vi "End Unpolled Mode.vi"(8 "error in":errorcluster, 11 "Neph in":refnum<class "Nephelometer.lvclass">) -> (0 "error out":errorcluster, 3 "Neph out":refnum<class "Nephelometer.lvclass">)   [LabVIEW 2014, in "Nephelometer.lvclass"]
uses:
  Nephelometer.lvclass
  Reusable/Session APIs/Serial/Serial Session.lvclass
  Nephelometer.lvclass/Nephelometer.ctl
  Accessors/Read Session Handle.vi
  <userlib>/_Session Fwk/Session - Root.lvclass
panel:
  out "Read - Asynchronous":string
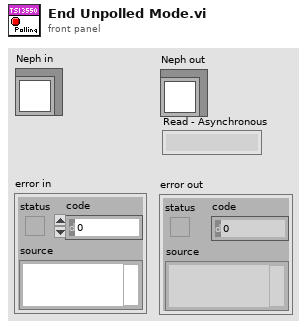
[diagram p1: front panel]
types:
  T1 = typedef "Session - Root.lvclass/Session Handle.ctl" = refnum<data-value>
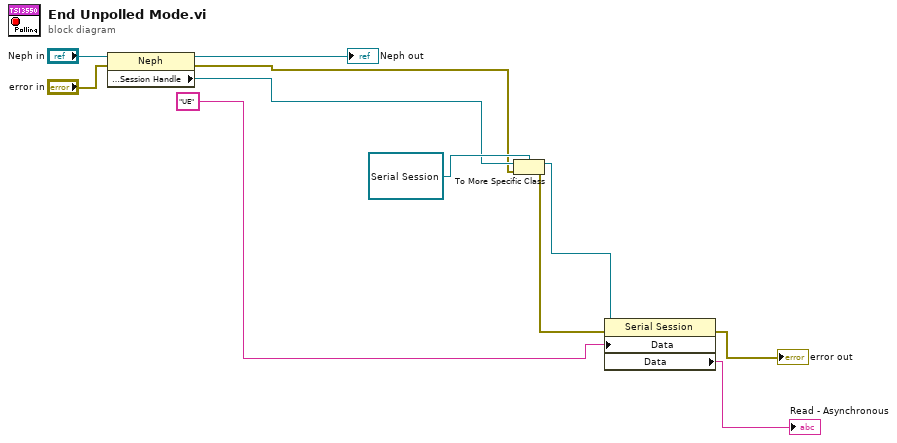
[diagram p0: block diagram]
diagram:
  n1 = property class="Neph"(reference="Neph in", error in="error in") -> (reference out=→"Neph out":refnum<class "Nephelometer.lvclass">, error out=w1:errorcluster, "Accessors:Session Handle"=w4:T1)
  n2 = To More Specific Class(target class=refnum<data-value> refnum ("Session Handle"), reference=w4, error in=w1) -> (specific class reference=w7:refnum<data-value>, error out=w6:errorcluster)
  n3 = property class="Serial Session"(reference=w7, error in=w6, "Data"="UE" ("Write - Asynchronous")) -> (error out=→"error out":errorcluster, "Data"=→"Read - Asynchronous":string)  [unwired: 1 out]
